vi "Get Core Plugin Settings.vi"(8 "error in (no error)":errorcluster, 11 "Item Ref in":T3 format="%.0x") -> (0 "error out":errorcluster, 2 "plugin configuration":T1={"name"="", "components"=[], "cycle timing"={"priority"=10000, "decimation"=1, "offset"=0}}, 3 "Item Ref out":T3 format="%.0x")   [LabVIEW 2021, in "DSF Shared.lvlib"]
uses:
  DSF Shared.lvlib
  <vilib>/NI VeriStand/Custom Device API/Custom Device API.lvlib
  <vilib>/NI VeriStand/Custom Device API/Get Item Property (Variant).vi
  Includes/DSF Core.lvlibp/Typedefs/DSF Timing Info.ctl
  Includes/DSF Core.lvlibp/Typedefs/Core Plugin Configuration.ctl
  <vilib>/NI VeriStand/Custom Device API/Custom Device Item Ref.ctl
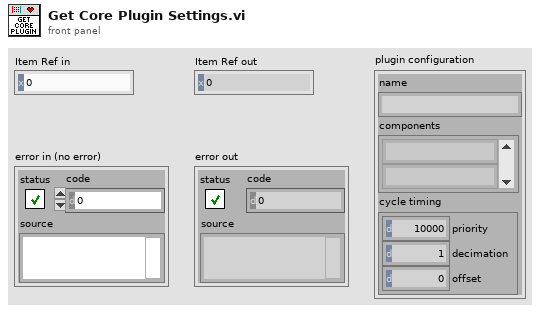
[diagram p1: front panel]
types:
  T1 = typedef "DSF Core.lvlibp/Plugin Configuration.lvclass/Core Plugin Configuration.ctl" = cluster{"name":string, "components":string[], "cycle timing":T2}
  T2 = typedef "DSF Core.lvlibp/DSF Timing Info.ctl" = cluster{"priority":u64, "decimation":u64, "offset":u64}
  T3 = typedef "Custom Device API.lvlib/Custom Device Item Ref.ctl" = u64
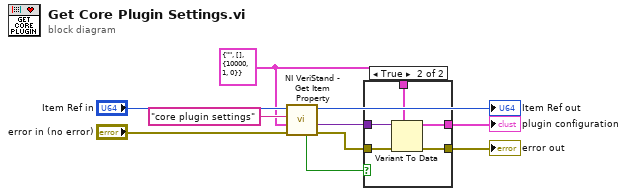
[diagram p0: block diagram]
diagram:
  w1 = T1 {"name"="", "components"=[], "cycle timing"={"priority"=10000, "decimation"=1, "offset"=0}} ("plugin configuration")
  n1 = call-poly <vilib>:"NI VeriStand - Get Item Property.vi"("error in (no error)"="error in (no error)", "Default Value"=w1, "Property Name"="core plugin settings" ("dsf options"), "Item Ref in"="Item Ref in") -> ("error out"=w9:errorcluster, "Value"=w8:variant, "Item Ref out"=→"Item Ref out":T3, "Found?"=w5:bool)  [unwired: 4 in]
  n2 = case shown="True" w5 {
    tunnel: w9 -> [w11 w17]
    tunnel: w1 -> [w12 w16]
    tunnel: w8 -> [_ w15]
    tunnel: [w11 w14] -> w7
    tunnel: [w12 w13] -> w3
    frame False {
    }
    frame True {
      n3 = Variant To Data(error in=w17, type=w16, Variant=w15) -> (data=w13:T1, error out=w14:errorcluster)
    }
  }
  "error out" <- w7
  "plugin configuration" <- w3
